vi "Get Term Em Variables.vi"(8 "error in (no error)":errorcluster, 11 "LabVIEW Web Service Request":refnum<class "Web Request.lvclass">) -> (0 "error out":errorcluster, 3 "LabVIEW Web Service Request out":refnum<class "Web Request.lvclass">)   [LabVIEW 2018]
doc: "This VI sets all of the ESP variables for a single contact so it can be output from an ESP script."
uses:
  <vilib>/wsapi/Web Request.lvclass
  CAEN globals.vi
  <vilib>/wsapi/class/subVIs/Set String ESP Variable.vi
panel:
  out "result string":string
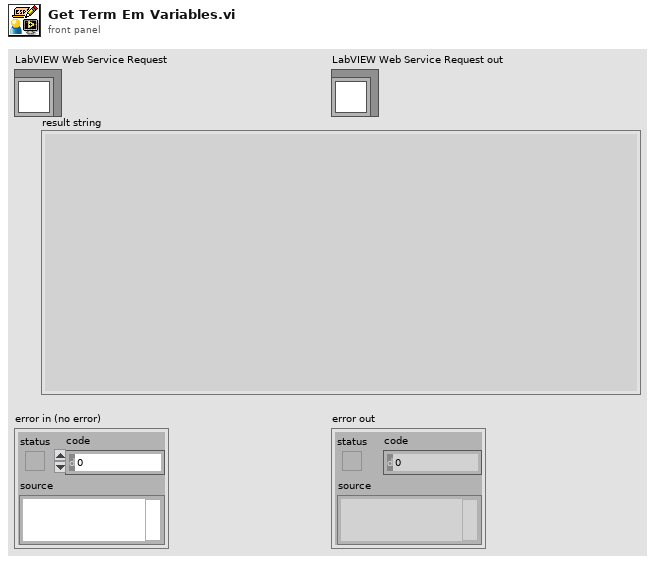
[diagram p1: front panel]
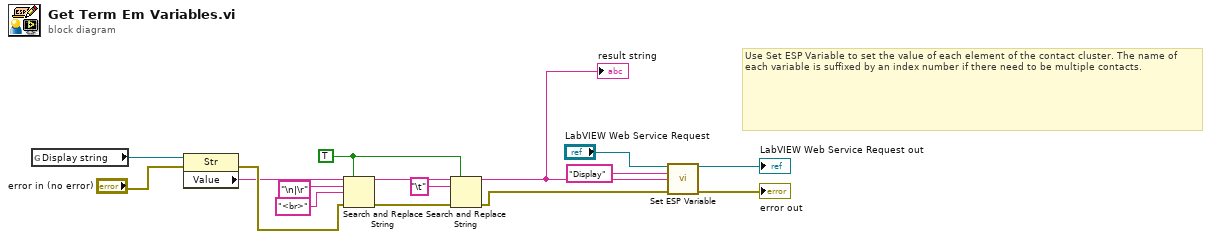
[diagram p0: block diagram]
diagram:
  w2 = TRUE ("replace all? (F)")
  # "Use Set ESP Variable to set the value of each element of the contact cluster. The name of each variable is suffixed by an index number if there need to be multiple contacts."
  n1 = global read "CAEN globals.vi" "Display string"() -> (w16:refnum<vi>)
  n2 = property class="Str"(reference=w16, error in="error in (no error)") -> (error out=w8:errorcluster, "Value"=w7:string)  [unwired: 1 out]
  n3 = Search and Replace String(replace all?=w2, input string=w7, search string="\n|\r", replace string="<br>" ("search string"), error in=w8) -> (result string=w4:string, error out=w6:errorcluster)  [unwired: 3 in, 2 out]
  n4 = Search and Replace String(replace all?=w2, input string=w4, search string="\t", error in=w6) -> (result string=w3:string, error out=w5:errorcluster)  [unwired: 4 in, 2 out]
  "result string" <- w3
  n5 = call-poly <vilib>:"Set ESP Variable.vi"("LabVIEW Web Service Request"="LabVIEW Web Service Request", "key"="Display" ("format string"), "value"=w3, "error in (no error)"=w5) -> ("LabVIEW Web Service Request out"=→"LabVIEW Web Service Request out":refnum<class "Web Request.lvclass">, "error out"=→"error out":errorcluster)  [unwired: 10 in]
